vi "RaiseError.vi"(8 "error in (no error)":errorcluster, 9 "Error Description":string, 10 "Error Title":string, 11 "Error Code":i32) -> (0 "error out":errorcluster)   [LabVIEW 2009, in "LD ErrorHandler.lvlib"]
doc: "Use this method to raise errors in LapDog source code or code that plugs into a LapDog component."
uses:
  LD ErrorHandler.lvlib
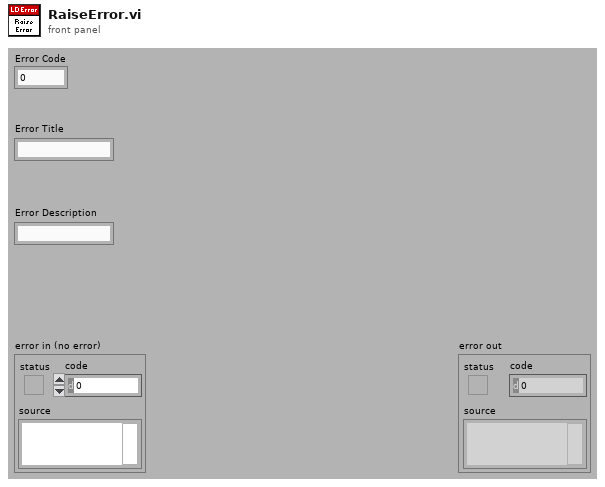
[diagram p1: front panel]
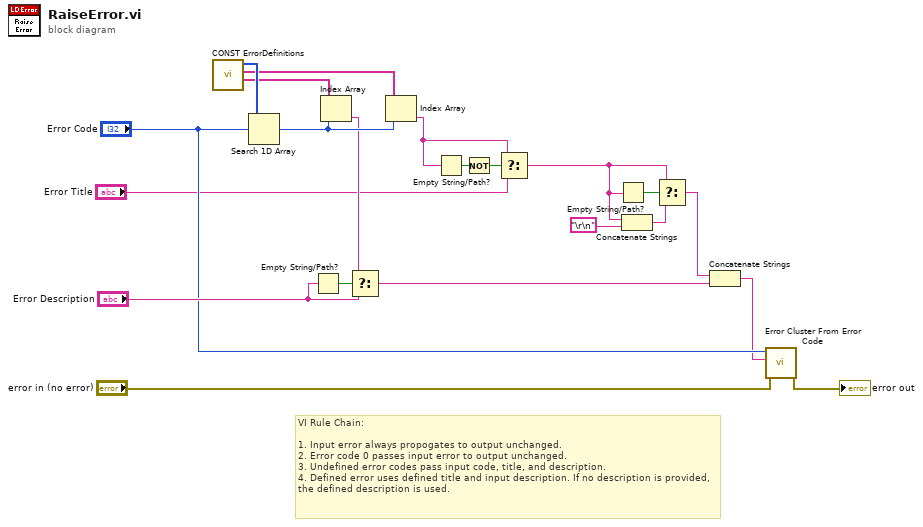
[diagram p0: block diagram]
diagram:
  # "VI Rule Chain:\n\n1. Input error always propogates to output unchanged.\n2. Error code 0 passes input error to output unchanged.\n3. Undefined error codes pass input code, title, and description.\n4. Defined error uses defined title and input description. If no description is provided, the defined description is used."
  n1 = call "CONST ErrorDefinitions.vi"() -> ("Error Descriptions"=w17:string[], "Error Titles"=w16:string[], "Error Codes"=w18:i32[])  [unwired: 9 in]
  n2 = Search 1D Array(1D array=w18, element="Error Code") -> (index of element=w13:i32)  [unwired: 1 in]
  n3 = Empty String/Path?(string/path="Error Description") -> (empty?=w11:bool)
  n4 = Index Array(array=w17, index=w13) -> (element=w12:string)
  n5 = Select(t=w12, s=w11, f="Error Description") -> (s? t:f=w10:string)
  n6 = Index Array(array=w16, index=w13) -> (element=w6:string)
  n7 = Empty String/Path?(string/path=w6) -> (empty?=w9:bool)
  n8 = Not(x=w9) -> (.not. x?=w8:bool)
  n9 = Select(t=w6, s=w8, f="Error Title") -> (s? t:f=w4:string)
  n10 = Empty String/Path?(string/path=w4) -> (empty?=w5:bool)
  n11 = Concatenate Strings(w4, "\r\n") -> (w2:string)
  n12 = Select(t=w4, s=w5, f=w2) -> (s? t:f=w1:string)
  n13 = Concatenate Strings(w1, w10) -> (w14:string)
  n14 = call "Error Cluster From Error Code.vi"("error in (no error)"="error in (no error)", "error message (\"\")"=w14, "error code (0)"="Error Code") -> ("error out"=→"error out":errorcluster)  [unwired: 6 in]
